vi "Process_2s_complement.vi"(0 "uC Raw data":u8[][](array[numeric])) -> (1 "Real Data":i32[](array[numeric]), 2 "Imag Data":i32[](array[numeric]))   [LabVIEW 2011, in "NMR.lvclass"]
uses:
  NMR.lvclass
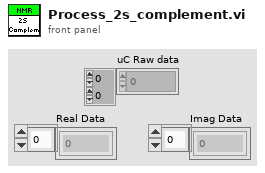
[diagram p1: front panel]
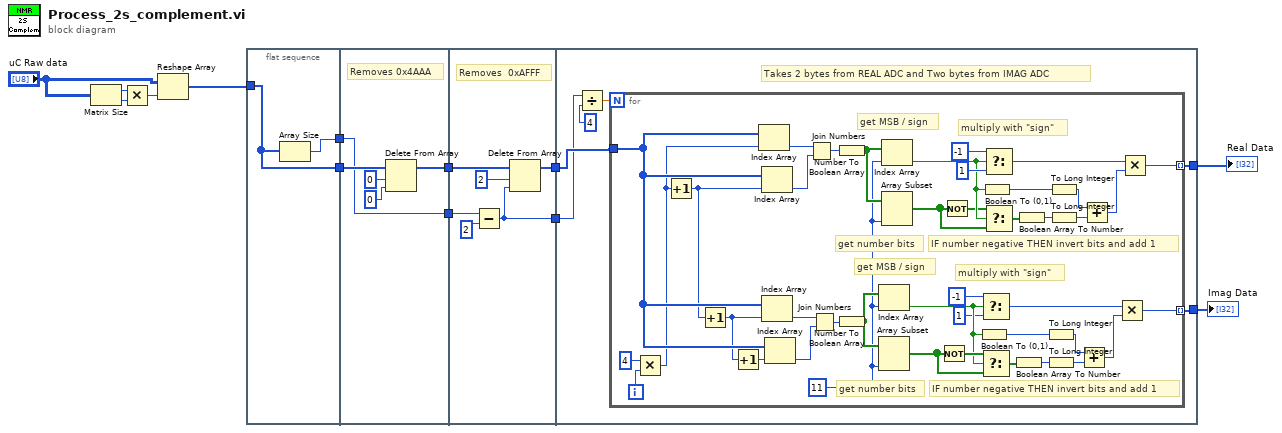
[diagram p0: block diagram]
diagram:
  n1 = Matrix Size(0:"uC Raw data") -> (1:w3:i32, 2:w2:i32)
  n2 = Multiply(x=w3, y=w2) -> (x*y=w4:i32)
  n3 = Reshape Array("uC Raw data", w4) -> (w5:u8[])
  n4 = flat-sequence {
    tunnel: [w15] -> w13
    tunnel: [w14] -> w12
    tunnel: w5 -> [w15]
    tunnel: w13 -> [w20]
    tunnel: w12 -> [w16]
    tunnel: [w18] -> w11
    tunnel: [w16] -> w10
    tunnel: w11 -> [w26]
    tunnel: w10 -> [w22]
    tunnel: [w24] -> w9
    tunnel: [w21] -> w8
    tunnel: w9 -> [w32]
    tunnel: [w31] -> w6
    tunnel: [w30] -> w7
    tunnel: w8 -> [w28]
    frame #0 {
      n5 = Array Size(array=w15) -> (size(s)=w14:i32)
    }
    frame #1 {
      # "Removes 0x4AAA"
      n6 = Delete From Array(array=w20, length=0, index=0) -> (array with subset deleted=w18:u8[])  [unwired: 1 out]
    }
    frame #2 {
      # "Removes  0xAFFF"
      n7 = Subtract(x=w22, y=2 ("length")) -> (x-y=w21:i32)
      n8 = Delete From Array(array=w26, length=2, index=w21) -> (array with subset deleted=w24:u8[])  [unwired: 1 out]
    }
    frame #3 {
      # "Takes 2 bytes from REAL ADC and Two bytes from IMAG ADC"
      n9 = Divide(x=w28, y=4) -> (x/y=w27:dbl)
      n10 = for {
        N: w27 -> [_]
        tunnel: w32 -> [w69]
        tunnel: [w48] -> w31 mode=indexing
        tunnel: [w34] -> w30 mode=indexing
        i -> [w66]
        w33 = 11 ("length")
        # "multiply with \"sign\""
        # "IF number negative THEN invert bits and add 1"
        # "get number bits"
        # "get MSB / sign"
        # "multiply with \"sign\""
        # "IF number negative THEN invert bits and add 1"
        # "get number bits"
        # "get MSB / sign"
        n11 = Multiply(x=4, y=w66) -> (x*y=w64:i32)
        n12 = Increment(x=w64) -> (x+1=w67:i32)
        n13 = Increment(x=w67) -> (x+1=w68:i32)
        n14 = Increment(x=w68) -> (x+1=w70:i32)
        n15 = Index Array(array=w69, index=w64) -> (element=w74:u8)
        n16 = Index Array(array=w69, index=w67) -> (element=w73:u8)
        n17 = Index Array(array=w69, index=w68) -> (element=w71:u8)
        n18 = Index Array(array=w69, index=w70) -> (element=w72:u8)
        n19 = Join Numbers(hi=w74, lo=w73) -> ((hi.lo)=w62:u16)
        n20 = Join Numbers(hi=w71, lo=w72) -> ((hi.lo)=w63:u16)
        n21 = Number To Boolean Array(number=w62) -> (Boolean array=w49:bool[])
        n22 = Number To Boolean Array(number=w63) -> (Boolean array=w35:bool[])
        n23 = Index Array(array=w35, index=w33) -> (element=w41:bool)
        n24 = Array Subset(array=w35, length=w33) -> (w45:bool[])  [unwired: 1 in]
        n25 = Index Array(array=w49, index=w33) -> (element=w56:bool)
        n26 = Array Subset(array=w49, length=w33) -> (w52:bool[])  [unwired: 1 in]
        n27 = Not(x=w45) -> (.not. x?=w46:bool[])
        n28 = Not(x=w52) -> (.not. x?=w51:bool[])
        n29 = Boolean To (0,1)(Boolean=w41) -> (0, 1=w42:i16)
        n30 = Select(t=-1, s=w41, f=1) -> (s? t:f=w38:i32)
        n31 = Select(t=w46, s=w41, f=w45) -> (s? t:f=w44:bool[])
        n32 = Boolean To (0,1)(Boolean=w56) -> (0, 1=w55:i16)
        n33 = Select(t=-1, s=w56, f=1) -> (s? t:f=w59:i32)
        n34 = Select(t=w51, s=w56, f=w52) -> (s? t:f=w53:bool[])
        n35 = Boolean Array To Number(Boolean array=w44) -> (number=w47:u32)
        n36 = Boolean Array To Number(Boolean array=w53) -> (number=w50:u32)
        n37 = To Long Integer(number=w42) -> (32bit integer=w36:i32)
        n38 = To Long Integer(number=w47) -> (32bit integer=w43:i32)
        n39 = To Long Integer(number=w55) -> (32bit integer=w61:i32)
        n40 = To Long Integer(number=w50) -> (32bit integer=w54:i32)
        n41 = Add(x=w36, y=w43) -> (x+y=w37:i32)
        n42 = Add(x=w61, y=w54) -> (x+y=w60:i32)
        n43 = Multiply(x=w38, y=w37) -> (x*y=w34:i32)
        n44 = Multiply(x=w59, y=w60) -> (x*y=w48:i32)
      }
    }
  }
  "Real Data" <- w6
  "Imag Data" <- w7
